vi "tdms.vi"() -> ()   [LabVIEW 2020]
uses:
  <vilib>/Utility/error.llb/DialogType.ctl
  <vilib>/Utility/TDMS File Viewer/NI_TDMS File Viewer.lvlib
panel:
  out "data":dbl[][](array[numeric])
  out "date":string
  in  "user":string
  out "Array":dbl[][](array[numeric])
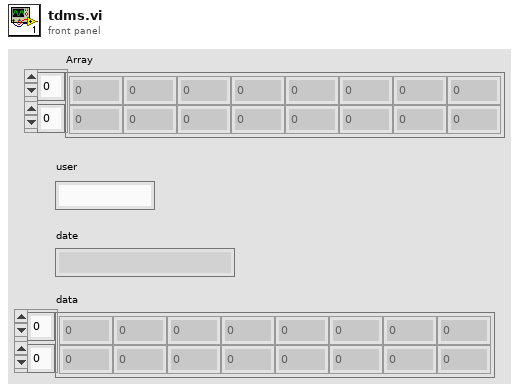
[diagram p1: front panel]
types:
  T1 = enum16{"open", "open or create", "create or replace", "create", "open (read-only)"}
  T2 = typedef "DialogType.ctl" = u16
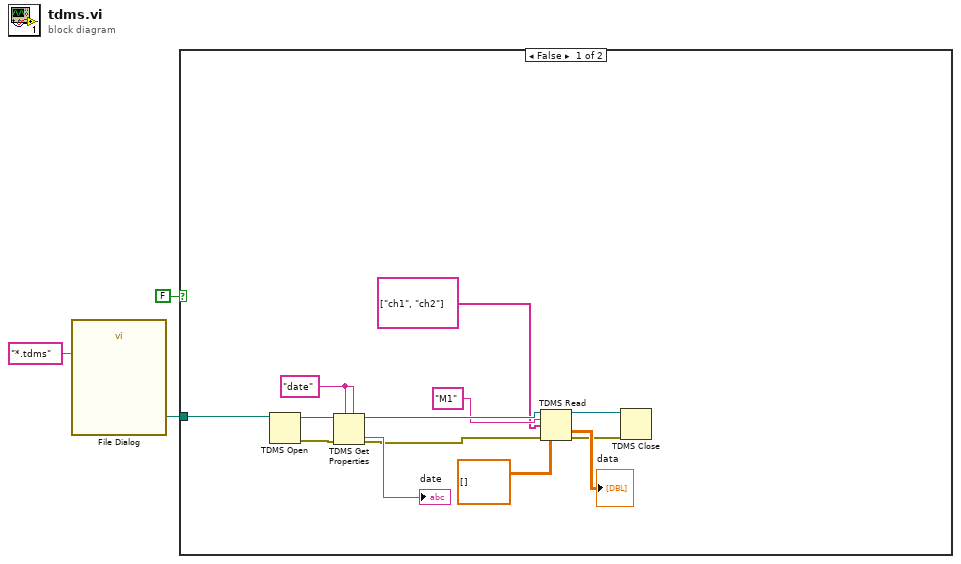
[diagram p0: block diagram]
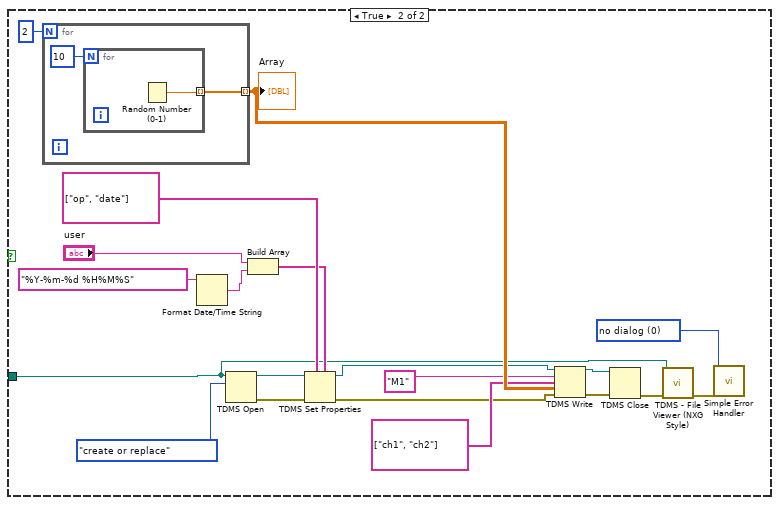
[diagram p2: hidden frame]
diagram:
  n1 = call "File Dialog"("pattern (all files)"="*.tdms") -> ("selected path"=w2:path)  [unwired: 11 in, 3 out]
  n2 = case shown="False" FALSE {
    tunnel: w2 -> [w16 w26]
    frame False {
      w13 = "date"
      n3 = TDMS Open(11:w16) -> (0:w14:errorcluster, 3:w15:refnum<k34>)  [unwired: 6 in]
      n4 = TDMS Get Properties(5:w13, 7:w13, 8:w14, 11:w15) -> (0:w10:errorcluster, 3:w11:refnum<k34>, 4:→"date":string)  [unwired: 2 in, 3 out]
      n5 = TDMS Read(0:w11, 5:"M1", 7:string[] ["ch1", "ch2"], 11:w10, 12:dbl[][] []) -> (4:w5:refnum<k34>, 10:→"data":dbl[][], 15:w4:errorcluster)  [unwired: 3 in, 3 out]
      n6 = TDMS Close(8:w4, 11:w5) -> ()  [unwired: 2 out]
    }
    frame True {
      w21 = T2 0 items=["no dialog", "OK message", "continue or stop message", "OK message + warnings", "continue/stop + warnings"] ("type of dialog (OK msg:1)")
      n7 = for {
        N: 2 -> [_]
        tunnel: [w37] -> w27 mode=indexing
        n8 = for {
          N: 10 -> [_]
          tunnel: [w39] -> w37 mode=indexing
          n9 = Random Number (0-1)() -> (number: 0 to 1=w39:dbl)
        }
      }
      "Array" <- w27
      n10 = Format Date/Time String(time format string (%c)="%Y-%m-%d %H%M%S") -> (date/time string=w29:string)  [unwired: 2 in]
      n11 = TDMS Open(10:T1."create or replace" ("operation (0:open)"), 11:w26) -> (0:w33:errorcluster, 3:w34:refnum<k34>)  [unwired: 5 in]
      n12 = Build Array("user", w29) -> (w28:string[])
      n13 = TDMS Set Properties(5:w28, 7:string[] ["op", "date"], 8:w33, 11:w34) -> (0:w17:errorcluster, 3:w18:refnum<k34>)  [unwired: 2 in, 2 out]
      n14 = TDMS Write(0:w18, 5:"M1", 7:string[] ["ch1", "ch2"], 9:w27, 11:w17) -> (4:w25:refnum<k34>, 15:w24:errorcluster)  [unwired: 1 in, 2 out]
      n15 = TDMS Close(8:w24, 11:w25) -> (0:w23:errorcluster)  [unwired: 1 out]
      n16 = call <vilib>:"TDMS - File Viewer (NXG Style).vi"("error in"=w23, "file in"=w26) -> ("error out"=w22:errorcluster)  [unwired: 8 in, 1 out]
      n17 = call <vilib>:"Simple Error Handler.vi"("type of dialog (OK msg:1)"=w21, "error in (no error)"=w22) -> ()  [unwired: 3 in, 5 out]
    }
  }
